vi "BioFeedback7(8-channelSubViewTo2DVR.vi"(0 "UI Data Right":path=path "C:/Users/Tinggroup/Desktop/VRMuscleActivationVisualizer/StationaryVisualFeedbackVR/assets/BiofeedbackData.txt", 7 "Frames Per Second":dbl=30.0, 9 "Start Trial":bool, 11 "End Trial":bool, 12 "Data Directory":path, 13 "File Name":string, 14 "Extension":string="_EMG.txt") -> ()   [LabVIEW 2016]
uses:
  <vilib>/Utility/error.llb/DialogType.ctl
  <vilib>/Analysis/5stat.llb/RMS (DBL).vi
  <vilib>/Waveform/WDTFileIO.llb/Export Waveform To Spreadsheet File.vi
  <vilib>/Waveform/WDTOps.llb/WDT Append Waveforms DBL.vi
  <vilib>/Analysis/NI_AALPro.lvlib
  <resource>/objmgr/daqmx.rc
panel:
  out "Target Graph":cluster{dbl[], dbl[]}(graph)
  in  "RightSignalB":dbl
  in  "RightSignalA":dbl
  in  "LefftSignalB":dbl
  in  "LeftSignalA":dbl
  out "Aggregate 8":waveform(dbl)[](array[waveform])
  in  "UI Data Left":path=path "C:/Users/Tinggroup/Desktop/VRMuscleActivationVisualizer/StationaryVisualFeedbackVR/assets/BiofeedbackData.txt"
  in  "EMG Input Device\nProduct Type":string
  out "Moving Avg Left":dbl(slide) scale=0.0..0.1
  out "Moving Avg Right":dbl(slide) scale=0.0..0.1
  out "RMS Right":dbl(graph)
  out "RMS Left":dbl(graph)
  out "RMS 8":dbl(graph)
  out "RMS 7":dbl(graph)
  out "RMS 6":dbl(graph)
  out "RMS 5":dbl(graph)
  out "RMS 4":dbl(graph)
  out "RMS 3":dbl(graph)
  out "RMS 2":dbl(graph)
  out "RMS 1":dbl(graph)
  out "Aggregate7":waveform(dbl)[](array[waveform])
  out "Aggregate6":waveform(dbl)[](array[waveform])
  out "Aggregate5":waveform(dbl)[](array[waveform])
  out "Aggregate4":waveform(dbl)[](array[waveform])
  out "Aggregate3":waveform(dbl)[](array[waveform])
  out "Aggregate2":waveform(dbl)[](array[waveform])
  out "Aggregate1":waveform(dbl)[](array[waveform])
  out "Wfm8":waveform(dbl)(graph)
  out "Wfm7":waveform(dbl)(graph)
  out "Wfm6":waveform(dbl)(graph)
  out "Wfm5":waveform(dbl)(graph)
  out "Wfm4":waveform(dbl)(graph)
  out "Wfm3":waveform(dbl)(graph)
  out "Wfm2":waveform(dbl)(graph)
  out "Wfm1":waveform(dbl)(graph)
  out "Trial Data":waveform(dbl)(graph)
  in  "UI Percent Path":path=path "C:/Users/Tinggroup/Desktop/VRMuscleActivationVisualizer/StationaryVisualFeedbackVR/assets/BiofeedbackTargetPercentage.txt"
  in  "Target Percentage":dbl=10.0
  out "Trial In Progress":bool
  in  "Trial Number":dbl
  in  "MARK":bool
  in  "Lower Cut-Off":dbl=20.0
  in  "Upper Cut-Off":dbl=300.0
  out "raw data":dynamicdata(graph)
  out "Bufffer Index":dbl
  out "Frames in Buffer":dbl
  out "Samples per frame":dbl
  out "Reset Data Acquisition\nAnd UI Updating":bool=TRUE
  in  "Moving Average Length (s)":dbl=0.5
  in  "Sample rate (Hz)":dbl=2000.0
  in  "End Program":bool
  # "Save Trial Data"
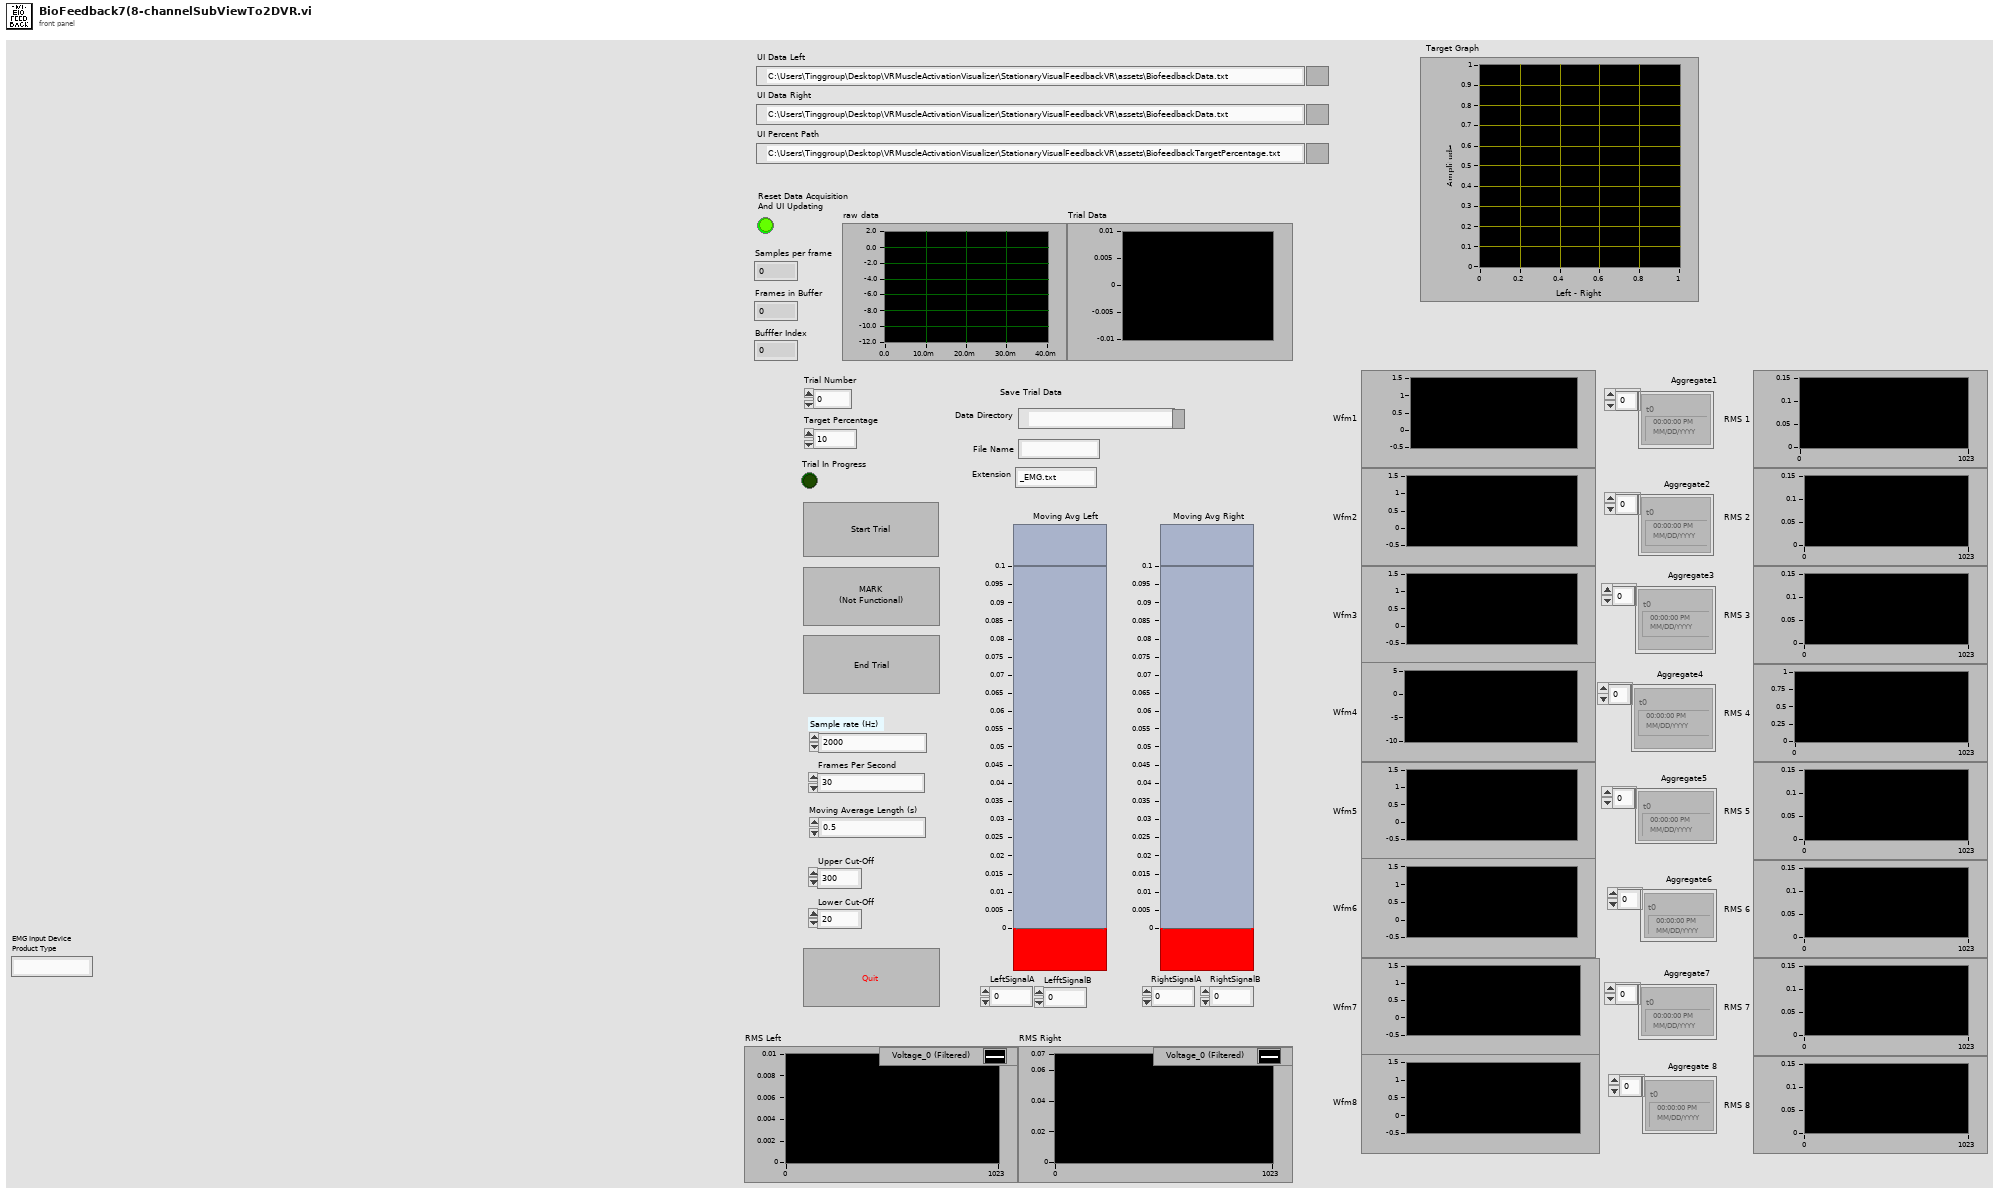
[diagram p1: front panel]
types:
  T1 = typedef "DialogType.ctl" = u16
  T2 = typedef "WaveformArrayControl.ctl" = waveform(dbl)[]
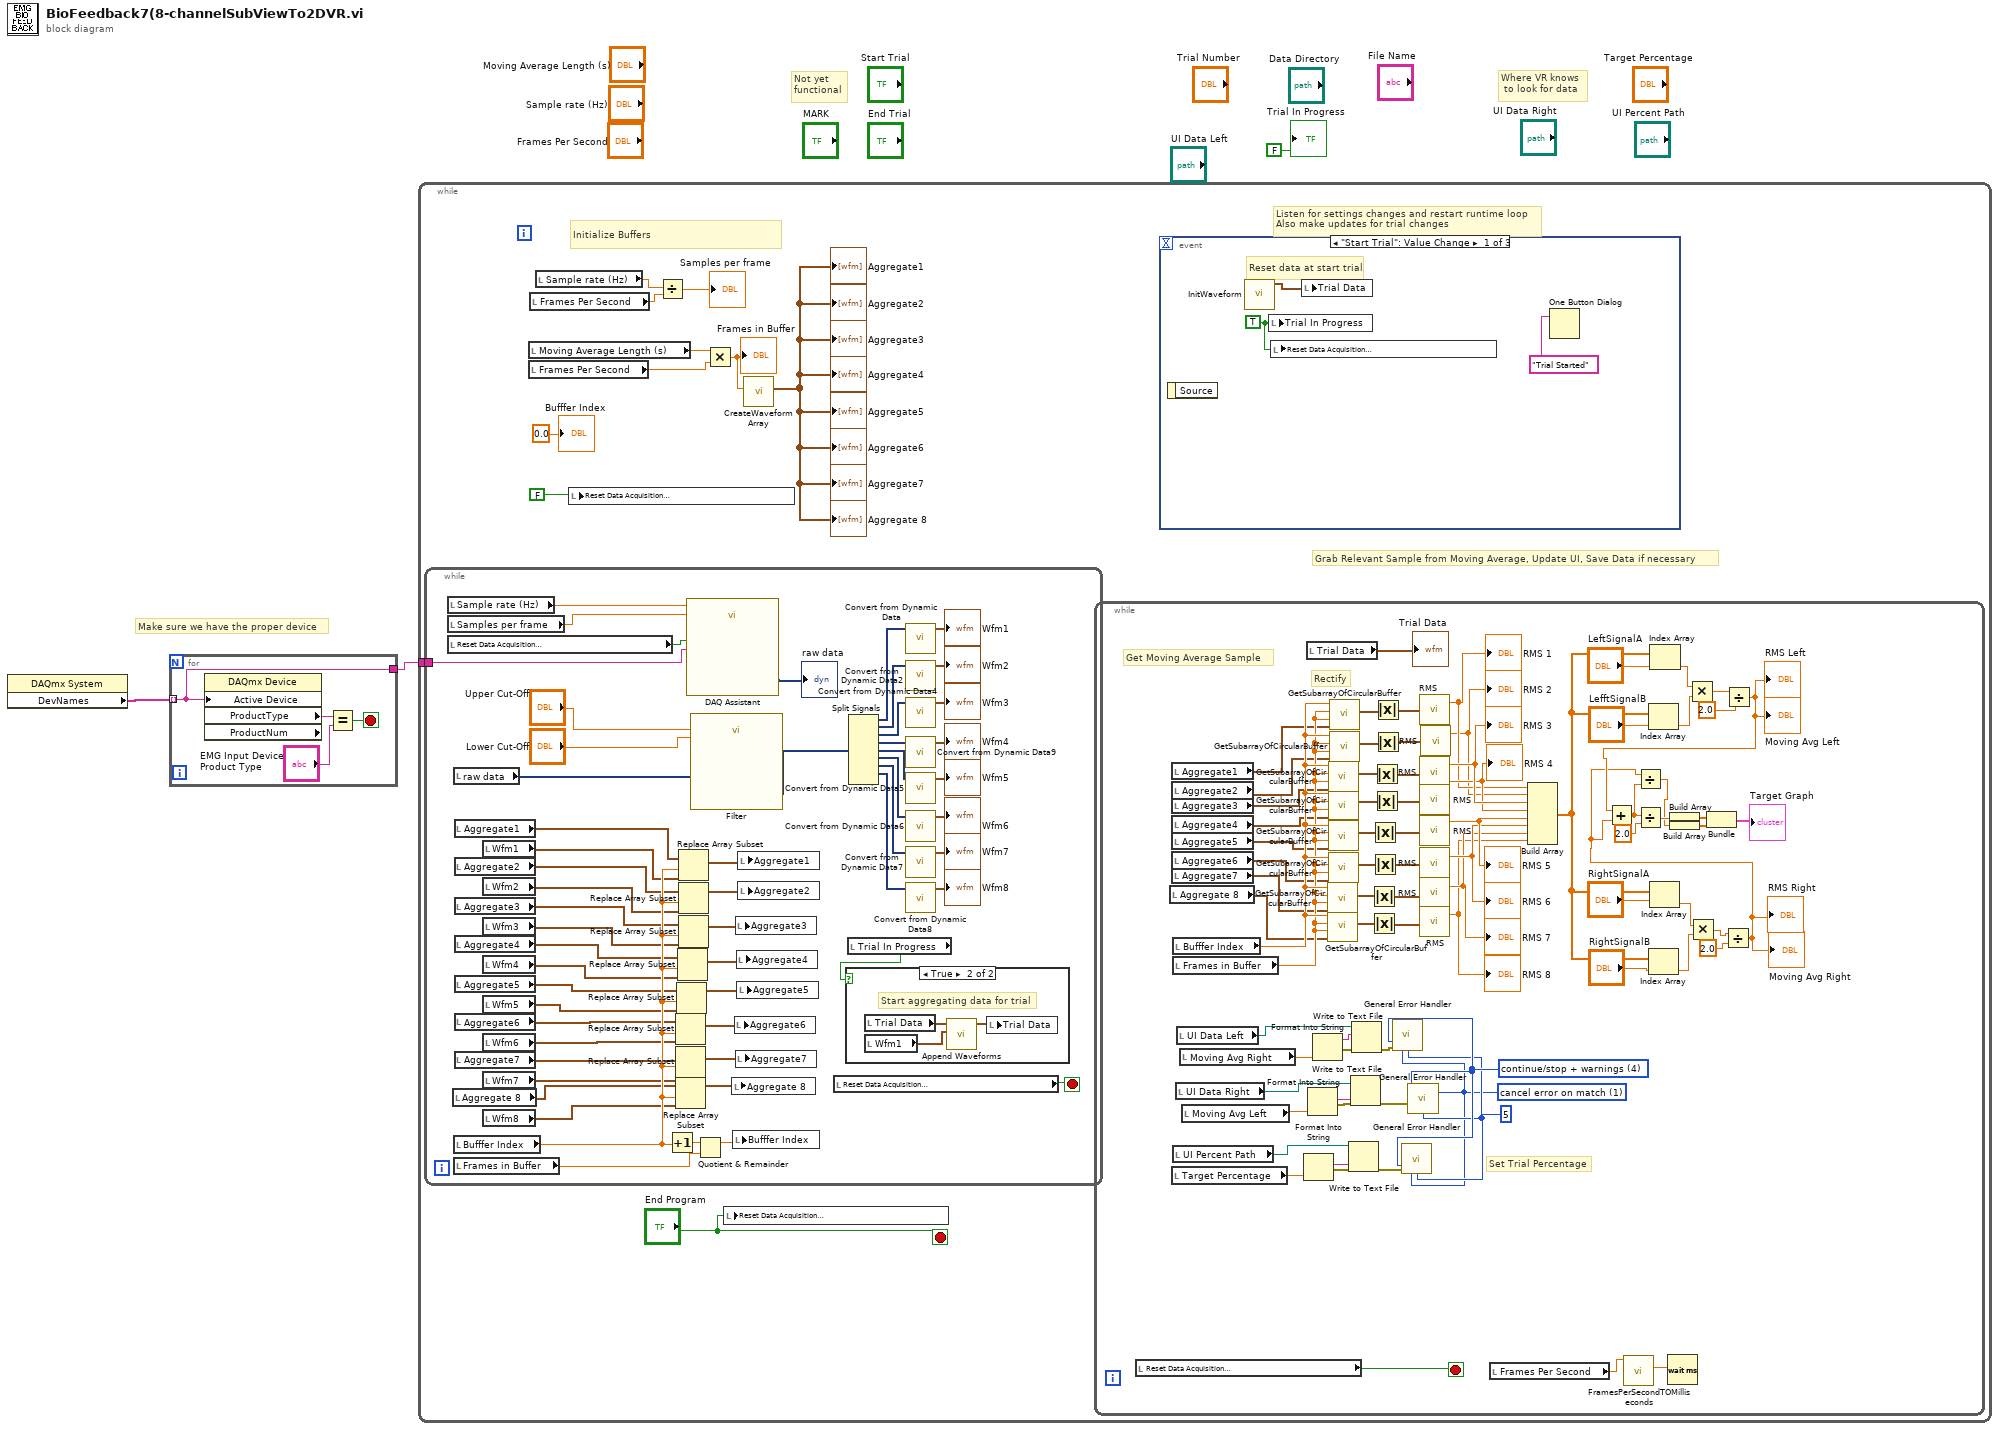
[diagram p0: block diagram]
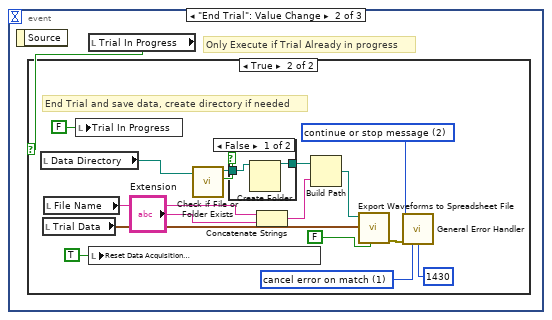
[diagram p2: hidden frame]
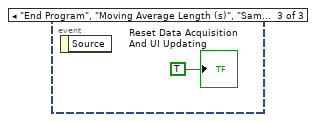
[diagram p5: hidden frame]
diagram:
  # "Make sure we have the proper device"
  # "Not yet \nfunctional"
  # "Where VR knows\n to look for data"
  n1 = property class="DAQmx System"() -> ("DevNames"=w2:tag[])  [unwired: 2 in, 2 out]
  n2 = for {
    tunnel: w2 -> [w4] mode=indexing
    tunnel: [w4] -> w1
    stop <- w5 stop-if-true
    n3 = property class="DAQmx Device" props=["Active Device", "ProductType", "ProductNum"]("Active Device"=w4) -> ("ProductType"=w7:string)  [unwired: 2 in, 3 out]
    n4 = Equal?(x=w7, y="EMG Input Device\nProduct Type") -> (x = y?=w5:bool)
  }
  n5 = while {
    tunnel: w1 -> [w9]
    stop <- "End Program" stop-if-true
    # "Grab Relevant Sample from Moving Average, Update UI, Save Data if necessary"
    # "Initialize Buffers"
    # "Listen for settings changes and restart runtime loop\nAlso make updates for trial changes"
    n6 = while {
      tunnel: w9 -> [w123]
      stop <- w167 stop-if-true
      n7 = local read "Sample rate (Hz)"() -> (w175:dbl)
      n8 = local read "Samples per frame"() -> (w174:dbl)
      n9 = local read "Reset Data Acquisition\nAnd UI Updating"() -> (w166:bool)
      n10 = local read "Aggregate 8"() -> (w121:waveform(dbl)[])
      n11 = local read "raw data"() -> (w172:dynamicdata)
      n12 = local read "Bufffer Index"() -> (w147:dbl)
      n13 = local read "Frames in Buffer"() -> (w169:dbl)
      n14 = local read "Aggregate1"() -> (w146:waveform(dbl)[])
      n15 = local read "Aggregate2"() -> (w144:waveform(dbl)[])
      n16 = local read "Aggregate3"() -> (w142:waveform(dbl)[])
      n17 = local read "Aggregate4"() -> (w140:waveform(dbl)[])
      n18 = local read "Aggregate5"() -> (w138:waveform(dbl)[])
      n19 = local read "Aggregate6"() -> (w136:waveform(dbl)[])
      n20 = local read "Aggregate7"() -> (w134:waveform(dbl)[])
      n21 = local read "Wfm1"() -> (w145:waveform(dbl))
      n22 = local read "Wfm2"() -> (w143:waveform(dbl))
      n23 = local read "Wfm3"() -> (w141:waveform(dbl))
      n24 = local read "Wfm4"() -> (w139:waveform(dbl))
      n25 = local read "Wfm5"() -> (w137:waveform(dbl))
      n26 = local read "Wfm6"() -> (w135:waveform(dbl))
      n27 = local read "Wfm7"() -> (w133:waveform(dbl))
      n28 = local read "Wfm8"() -> (w132:waveform(dbl))
      n29 = Increment(x=w147) -> (x+1=w168:dbl)
      n30 = Replace Array Subset(array=w136, new element=w135, index=w147) -> (w126:waveform(dbl)[])
      n31 = Replace Array Subset(array=w134, new element=w133, index=w147) -> (w125:waveform(dbl)[])
      n32 = Replace Array Subset(array=w121, new element=w132, index=w147) -> (w122:waveform(dbl)[])
      n33 = Replace Array Subset(array=w138, new element=w137, index=w147) -> (w127:waveform(dbl)[])
      n34 = Replace Array Subset(array=w140, new element=w139, index=w147) -> (w128:waveform(dbl)[])
      n35 = Replace Array Subset(array=w146, new element=w145, index=w147) -> (w131:waveform(dbl)[])
      n36 = Replace Array Subset(array=w144, new element=w143, index=w147) -> (w130:waveform(dbl)[])
      n37 = Replace Array Subset(array=w142, new element=w141, index=w147) -> (w129:waveform(dbl)[])
      n38 = call "DAQ Assistant"("rate"=w175, "number of samples"=w174, "stop (T)"=w166, "device name"=w123) -> ("data"=→"raw data":dynamicdata)  [unwired: 13 in, 2 out]
      n39 = call "Filter"("Lower Cut-Off"="Lower Cut-Off", "Upper Cut-Off"="Upper Cut-Off", "Signal"=w172) -> ("Filtered Signal"=w164:dynamicdata)  [unwired: 7 in, 1 out]
      n40 = Quotient & Remainder(x=w168, y=w169) -> (x-y*floor(x/y)=w170:dbl)  [unwired: 1 out]
      n41 = local write "Aggregate 8"(w122) -> ()
      n42 = local write "Bufffer Index"(w170) -> ()
      n43 = local write "Aggregate6"(w126) -> ()
      n44 = local write "Aggregate3"(w129) -> ()
      n45 = local write "Aggregate7"(w125) -> ()
      n46 = local write "Aggregate4"(w128) -> ()
      n47 = local write "Aggregate5"(w127) -> ()
      n48 = local write "Aggregate1"(w131) -> ()
      n49 = local write "Aggregate2"(w130) -> ()
      n50 = local read "Reset Data Acquisition\nAnd UI Updating"() -> (w167:bool)
      n51 = local read "Trial In Progress"() -> (w124:bool)
      n52 = case shown="True" w124 {
        frame False {
        }
        frame True {
          # "Start aggregating data for trial"
          n53 = local read "Trial Data"() -> (w178:waveform(dbl))
          n54 = local read "Wfm1"() -> (w177:waveform(dbl))
          n55 = call-poly <vilib>:"Append Waveforms.vi"("waveform B"=w177, "waveform A"=w178) -> ("waveform out"=w176:waveform(dbl))  [unwired: 8 in, 1 out]
          n56 = local write "Trial Data"(w176) -> ()
        }
      }
      n57 = Split Signals(w164) -> (w163:dynamicdata, w162:dynamicdata, w161:dynamicdata, w160:dynamicdata, w159:dynamicdata, w158:dynamicdata, w157:dynamicdata, w156:dynamicdata)  [unwired: 9 in, 1 out]
      n58 = call "Convert from Dynamic Data"("Dynamic Data Type"=w163) -> ("Waveform"=→"Wfm1":waveform(dbl))  [unwired: 3 in]
      n59 = call "Convert from Dynamic Data2"("Dynamic Data Type"=w162) -> ("Waveform"=→"Wfm2":waveform(dbl))  [unwired: 3 in]
      n60 = call "Convert from Dynamic Data4"("Dynamic Data Type"=w161) -> ("Waveform"=→"Wfm3":waveform(dbl))  [unwired: 3 in]
      n61 = call "Convert from Dynamic Data9"("Dynamic Data Type"=w160) -> ("Waveform"=→"Wfm4":waveform(dbl))  [unwired: 3 in]
      n62 = call "Convert from Dynamic Data5"("Dynamic Data Type"=w159) -> ("Waveform"=→"Wfm5":waveform(dbl))  [unwired: 3 in]
      n63 = call "Convert from Dynamic Data6"("Dynamic Data Type"=w158) -> ("Waveform"=→"Wfm6":waveform(dbl))  [unwired: 3 in]
      n64 = call "Convert from Dynamic Data7"("Dynamic Data Type"=w157) -> ("Waveform"=→"Wfm7":waveform(dbl))  [unwired: 3 in]
      n65 = call "Convert from Dynamic Data8"("Dynamic Data Type"=w156) -> ("Waveform"=→"Wfm8":waveform(dbl))  [unwired: 3 in]
    }
    n66 = local read "Moving Average Length (s)"() -> (w15:dbl)
    n67 = local read "Frames Per Second"() -> (w14:dbl)
    n68 = local read "Frames Per Second"() -> (w17:dbl)
    n69 = local read "Sample rate (Hz)"() -> (w18:dbl)
    n70 = local write "Reset Data Acquisition\nAnd UI Updating"(FALSE) -> ()
    n71 = Divide(x=w18, y=w17) -> (x/y=→"Samples per frame":dbl)
    n72 = Multiply(x=w15, y=w14) -> (x*y=w11:dbl)
    "Frames in Buffer" <- w11
    n73 = local write "Reset Data Acquisition\nAnd UI Updating"("End Program") -> ()
    n74 = call "CreateWaveformArray.vi"("bufferSize"=w11) -> ("initialized array"=→"Aggregate1" →"Aggregate2" →"Aggregate3" →"Aggregate4" →"Aggregate5" →"Aggregate6" →"Aggregate7" →"Aggregate 8":waveform(dbl)[])  [unwired: 5 in, 1 out]
    n75 = while {
      stop <- w120 stop-if-true
      w75 = T1 4 items=["no dialog", "OK message", "continue or stop message", "OK message + warnings", "continue/stop + warnings"] ("type of dialog (OK msg:1)")
      w73 = 1 items=["no exception", "cancel error on match", "set error on match"] ("[exception action] (none:0)")
      w74 = 5 ("[exception code]")
      # "Set Trial Percentage"
      # "Get Moving Average Sample"
      # "Rectify"
      n76 = local read "Reset Data Acquisition\nAnd UI Updating"() -> (w120:bool)
      n77 = local read "Aggregate 8"() -> (w72:waveform(dbl)[])
      n78 = local read "Aggregate1"() -> (w109:waveform(dbl)[])
      n79 = local read "Aggregate2"() -> (w105:waveform(dbl)[])
      n80 = local read "Aggregate3"() -> (w108:waveform(dbl)[])
      n81 = local read "Aggregate4"() -> (w104:waveform(dbl)[])
      n82 = local read "Aggregate5"() -> (w107:waveform(dbl)[])
      n83 = local read "Aggregate6"() -> (w106:waveform(dbl)[])
      n84 = local read "Aggregate7"() -> (w103:waveform(dbl)[])
      n85 = local read "Target Percentage"() -> (w76:dbl)
      n86 = local read "Bufffer Index"() -> (w111:dbl)
      n87 = local read "Frames in Buffer"() -> (w110:dbl)
      n88 = local read "UI Percent Path"() -> (w77:path)
      n89 = local read "UI Data Right"() -> (w115:path)
      n90 = local read "UI Data Left"() -> (w83:path)
      n91 = local read "Moving Avg Right"() -> (w85:dbl)
      n92 = local read "Moving Avg Left"() -> (w113:dbl)
      n93 = Format Into String(w76) -> (resulting string=w78:string, error out=w79:errorcluster)  [unwired: 3 in]
      n94 = local read "Trial Data"() -> (→"Trial Data":waveform(dbl))
      n95 = Format Into String(w113) -> (resulting string=w114:string, error out=w116:errorcluster)  [unwired: 3 in]
      n96 = Format Into String(w85) -> (resulting string=w82:string, error out=w84:errorcluster)  [unwired: 3 in]
      n97 = call "GetSubarrayOfCircularBuffer.vi"("initialized array"=w103, "buffer size"=w110, "subset size"=w110, "start index"=w111) -> ("initialized array 2"=w96:T2)  [unwired: 7 in]
      n98 = call "GetSubarrayOfCircularBuffer.vi"("initialized array"=w72, "buffer size"=w110, "subset size"=w110, "start index"=w111) -> ("initialized array 2"=w95:T2)  [unwired: 7 in]
      n99 = call "GetSubarrayOfCircularBuffer.vi"("initialized array"=w108, "buffer size"=w110, "subset size"=w110, "start index"=w111) -> ("initialized array 2"=w100:T2)  [unwired: 7 in]
      n100 = call "GetSubarrayOfCircularBuffer.vi"("initialized array"=w104, "buffer size"=w110, "subset size"=w110, "start index"=w111) -> ("initialized array 2"=w99:T2)  [unwired: 7 in]
      n101 = call "GetSubarrayOfCircularBuffer.vi"("initialized array"=w107, "buffer size"=w110, "subset size"=w110, "start index"=w111) -> ("initialized array 2"=w98:T2)  [unwired: 7 in]
      n102 = call "GetSubarrayOfCircularBuffer.vi"("initialized array"=w106, "buffer size"=w110, "subset size"=w110, "start index"=w111) -> ("initialized array 2"=w97:T2)  [unwired: 7 in]
      n103 = call "GetSubarrayOfCircularBuffer.vi"("initialized array"=w109, "buffer size"=w110, "subset size"=w110, "start index"=w111) -> ("initialized array 2"=w102:T2)  [unwired: 7 in]
      n104 = call "GetSubarrayOfCircularBuffer.vi"("initialized array"=w105, "buffer size"=w110, "subset size"=w110, "start index"=w111) -> ("initialized array 2"=w101:T2)  [unwired: 7 in]
      n105 = Write to Text File(file (use dialog)=w77, text=w78, error in=w79) -> (error out=w80:errorcluster)  [unwired: 1 in, 2 out]
      n106 = Write to Text File(file (use dialog)=w115, text=w114, error in=w116) -> (error out=w117:errorcluster)  [unwired: 1 in, 2 out]
      n107 = Write to Text File(file (use dialog)=w83, text=w82, error in=w84) -> (error out=w81:errorcluster)  [unwired: 1 in, 2 out]
      n108 = Absolute Value(x=w96) -> (abs(x)=w89:T2)
      n109 = Absolute Value(x=w95) -> (abs(x)=w88:T2)
      n110 = Absolute Value(x=w98) -> (abs(x)=w91:T2)
      n111 = Absolute Value(x=w97) -> (abs(x)=w90:T2)
      n112 = Absolute Value(x=w100) -> (abs(x)=w93:T2)
      n113 = Absolute Value(x=w99) -> (abs(x)=w92:T2)
      n114 = Absolute Value(x=w102) -> (abs(x)=w94:T2)
      n115 = Absolute Value(x=w101) -> (abs(x)=w71:T2)
      n116 = call <vilib>:"General Error Handler.vi"("type of dialog (OK msg:1)"=w75, "error in (no error)"=w81, "[exception action] (none:0)"=w73, "[exception code]"=w74) -> ()  [unwired: 7 in, 5 out]
      n117 = call <vilib>:"General Error Handler.vi"("type of dialog (OK msg:1)"=w75, "error in (no error)"=w80, "[exception action] (none:0)"=w73, "[exception code]"=w74) -> ()  [unwired: 7 in, 5 out]
      n118 = call <vilib>:"General Error Handler.vi"("type of dialog (OK msg:1)"=w75, "error in (no error)"=w117, "[exception action] (none:0)"=w73, "[exception code]"=w74) -> ()  [unwired: 7 in, 5 out]
      n119 = call-poly <vilib>:"RMS.vi"("X"=w94) -> ("rms value"=w65:dbl)  [unwired: 1 out]
      "RMS 1" <- w65
      n120 = call-poly <vilib>:"RMS.vi"("X"=w93) -> ("rms value"=w70:dbl)  [unwired: 1 out]
      "RMS 3" <- w70
      n121 = call-poly <vilib>:"RMS.vi"("X"=w92) -> ("rms value"=w69:dbl)  [unwired: 1 out]
      "RMS 4" <- w69
      n122 = call-poly <vilib>:"RMS.vi"("X"=w91) -> ("rms value"=w68:dbl)  [unwired: 1 out]
      "RMS 5" <- w68
      n123 = call-poly <vilib>:"RMS.vi"("X"=w90) -> ("rms value"=w67:dbl)  [unwired: 1 out]
      "RMS 6" <- w67
      n124 = call-poly <vilib>:"RMS.vi"("X"=w89) -> ("rms value"=w66:dbl)  [unwired: 1 out]
      "RMS 7" <- w66
      n125 = call-poly <vilib>:"RMS.vi"("X"=w88) -> ("rms value"=w63:dbl)  [unwired: 1 out]
      "RMS 8" <- w63
      n126 = call-poly <vilib>:"RMS.vi"("X"=w71) -> ("rms value"=w64:dbl)  [unwired: 1 out]
      "RMS 2" <- w64
      n127 = local read "Frames Per Second"() -> (w119:dbl)
      n128 = Build Array(w65, w64, w70, w69, w68, w67, w66, w63) -> (w56:dbl[])
      n129 = call "FramesPerSecondTOMilliseconds.vi"("Thermometer\nFps"=w119) -> ("x*y"=w118:dbl)  [unwired: 10 in]
      n130 = Index Array(array=w56, index="LefftSignalB") -> (element=w60:dbl)
      n131 = Index Array(array=w56, index="RightSignalB") -> (element=w54:dbl)
      n132 = Index Array(array=w56, index="RightSignalA") -> (element=w55:dbl)
      n133 = Index Array(array=w56, index="LeftSignalA") -> (element=w59:dbl)
      n134 = Wait (ms)(milliseconds to wait=w118) -> ()  [unwired: 1 out]
      n135 = Multiply(x=w59, y=w60) -> (x*y=w87:dbl)
      n136 = Multiply(x=w55, y=w54) -> (x*y=w52:dbl)
      n137 = Divide(x=w52, y=2.0) -> (x/y=w43:dbl)
      "RMS Right" <- w43
      "Moving Avg Right" <- w43
      n138 = Divide(x=w87, y=2.0) -> (x/y=w44:dbl)
      "RMS Left" <- w44
      "Moving Avg Left" <- w44
      n139 = Add(x=w44, y=w43) -> (x+y=w48:dbl)
      n140 = Divide(x=w43, y=w48) -> (x/y=w47:dbl)
      n141 = Divide(x=w48, y=2.0) -> (x/y=w50:dbl)
      n142 = Build Array(w50) -> (w49:dbl[])
      n143 = Build Array(w47) -> (w46:dbl[])
      n144 = Bundle(w49, w46) -> (→"Target Graph":cluster{dbl[], dbl[]})  [unwired: 1 in]
    }
    n145 = event shown="[0] \"Start Trial\": Value Change" {
      selector: _ -> [_ _ _]
      dyn-events: _ -> [_ _ _]
      timeout: _ -> [_ _ _]
      event "Start Trial": Value Change {
        w20 = TRUE ("Trial In Progress")
        # "Reset data at start trial"
        n146 = event-data() -> ()  [unwired: 1 in, 1 out]
        n147 = call "InitWaveform.vi"() -> ("output waveform"=w21:waveform(dbl))  [unwired: 11 in]
        n148 = local write "Trial In Progress"(w20) -> ()
        n149 = local write "Reset Data Acquisition\nAnd UI Updating"(w20) -> ()
        n150 = local write "Trial Data"(w21) -> ()
        n151 = One Button Dialog(message="Trial Started") -> ()  [unwired: 1 in, 1 out]
      }
      event "End Trial": Value Change {
        # "Only Execute if Trial Already in progress"
        n152 = event-data() -> ()  [unwired: 1 in, 1 out]
        n153 = local read "Trial In Progress"() -> (w22:bool)
        n154 = case shown="True" w22 {
          frame False {
          }
          frame True {
            w31 = T1 2 items=["no dialog", "OK message", "continue or stop message", "OK message + warnings", "continue/stop + warnings"] ("type of dialog (OK msg:1)")
            w32 = 1 items=["no exception", "cancel error on match", "set error on match"] ("[exception action] (none:0)")
            # "End Trial and save data, create directory if needed"
            n155 = local read "Data Directory"() -> (w34:path)
            n156 = local read "Trial Data"() -> (w26:waveform(dbl))
            n157 = local read "File Name"() -> (w29:string)
            n158 = local write "Trial In Progress"(FALSE ("Trial In Progress")) -> ()
            n159 = local write "Reset Data Acquisition\nAnd UI Updating"(TRUE ("Reset Data Acquisition\nAnd UI Updating")) -> ()
            n160 = call <vilib>:"Check if File or Folder Exists.vi"("path"=w34) -> ("file or folder exists?"=w36:bool, "dup path"=w35:path)  [unwired: 8 in, 1 out]
            n161 = case shown="False" w36 {
              tunnel: [w39 w41] -> w27
              tunnel: w35 -> [w40 w41]
              frame False {
                n162 = Create Folder(path (use dialog)=w40) -> (created path=w39:path)  [unwired: 2 in, 2 out]
              }
              frame True {
              }
            }
            n163 = Concatenate Strings(w29, "Extension") -> (w28:string)
            n164 = Build Path(base path=w27, name or relative path=w28) -> (appended path=w25:path)
            n165 = call-poly <vilib>:"Export Waveforms to Spreadsheet File.vi"("append to file? (new file:F)"=FALSE, "waveform"=w26, "file path (dialog if empty)"=w25) -> ("error out"=w24:errorcluster)  [unwired: 7 in, 1 out]
            n166 = call <vilib>:"General Error Handler.vi"("type of dialog (OK msg:1)"=w31, "error in (no error)"=w24, "[exception action] (none:0)"=w32, "[exception code]"=1430) -> ()  [unwired: 7 in, 5 out]
          }
        }
      }
      event "End Program", "Moving Average Length (s)", "Sample rate (Hz)", "Frames Per Second": Value Change {
        n167 = event-data() -> ()  [unwired: 1 in, 1 out]
        "Reset Data Acquisition\nAnd UI Updating" <- TRUE
      }
    }
    "Bufffer Index" <- 0.0 ("Bufffer Index")
  }
  "Trial In Progress" <- FALSE ("Trial In Progress")
